vi "电信1801-2018012704-杜兴安-虚拟仪器作业3.vi"() -> ()   [LabVIEW 2020]
uses:
  <vilib>/Native 3D Graph/xcontrol/3DPC_SurfacePlot.xctl
  <vilib>/Waveform/DWDTOps.llb/DWDT Binary U32 to Digital.vi
  <vilib>/Analysis/NI_AALBase.lvlib
  <vilib>/Native 3D Graph/classes/Base Datatype.lvclass
panel:
  out "3D Graph 7":refnum<class "Base Datatype.lvclass">[](xcontrol) caption="三维图形"
  out "波形图表 2":dbl[][](graph)
  out "数字波形图 2":digitalwaveform(graph)
  out "3D Graph 4":refnum<class "Base Datatype.lvclass">[](xcontrol) caption="三维图形"
  out "强度图 2":dbl[][](graph)
  out "XY图 2":cluster{dbl[], dbl[]}(graph)
  in  "界限值":dbl
  out "报警tip":bool
  out "温度计1":dbl(slide) scale=0.0..100.0
  in  "停止 3":bool
  out "电压显示":dbl
  in  "电压表":dbl(knob) scale=0.0..10.0
  in  "停止 2":bool
  out "波形图表":dbl[][](graph)
  out "数字波形图":digitalwaveform(graph)
  out "3D Graph 3":refnum<class "Base Datatype.lvclass">[](xcontrol) caption="三维图形"
  out "3D Graph 2":refnum<class "Base Datatype.lvclass">[](xcontrol) caption="三维图形"
  out "3D Graph":refnum<class "Base Datatype.lvclass">[](xcontrol) caption="三维图形"
  out "强度图":dbl[][](graph)
  out "XY图":cluster{dbl[], dbl[]}(graph)
  in  "?":bool
  out "报警提示":bool
  out "温度计":dbl(slide) scale=0.0..100.0
  in  "温度报警限值":dbl
  in  "电压表(V)":dbl(knob) scale=0.0..10.0
  out "电压值(V)":dbl
  in  "停止":bool
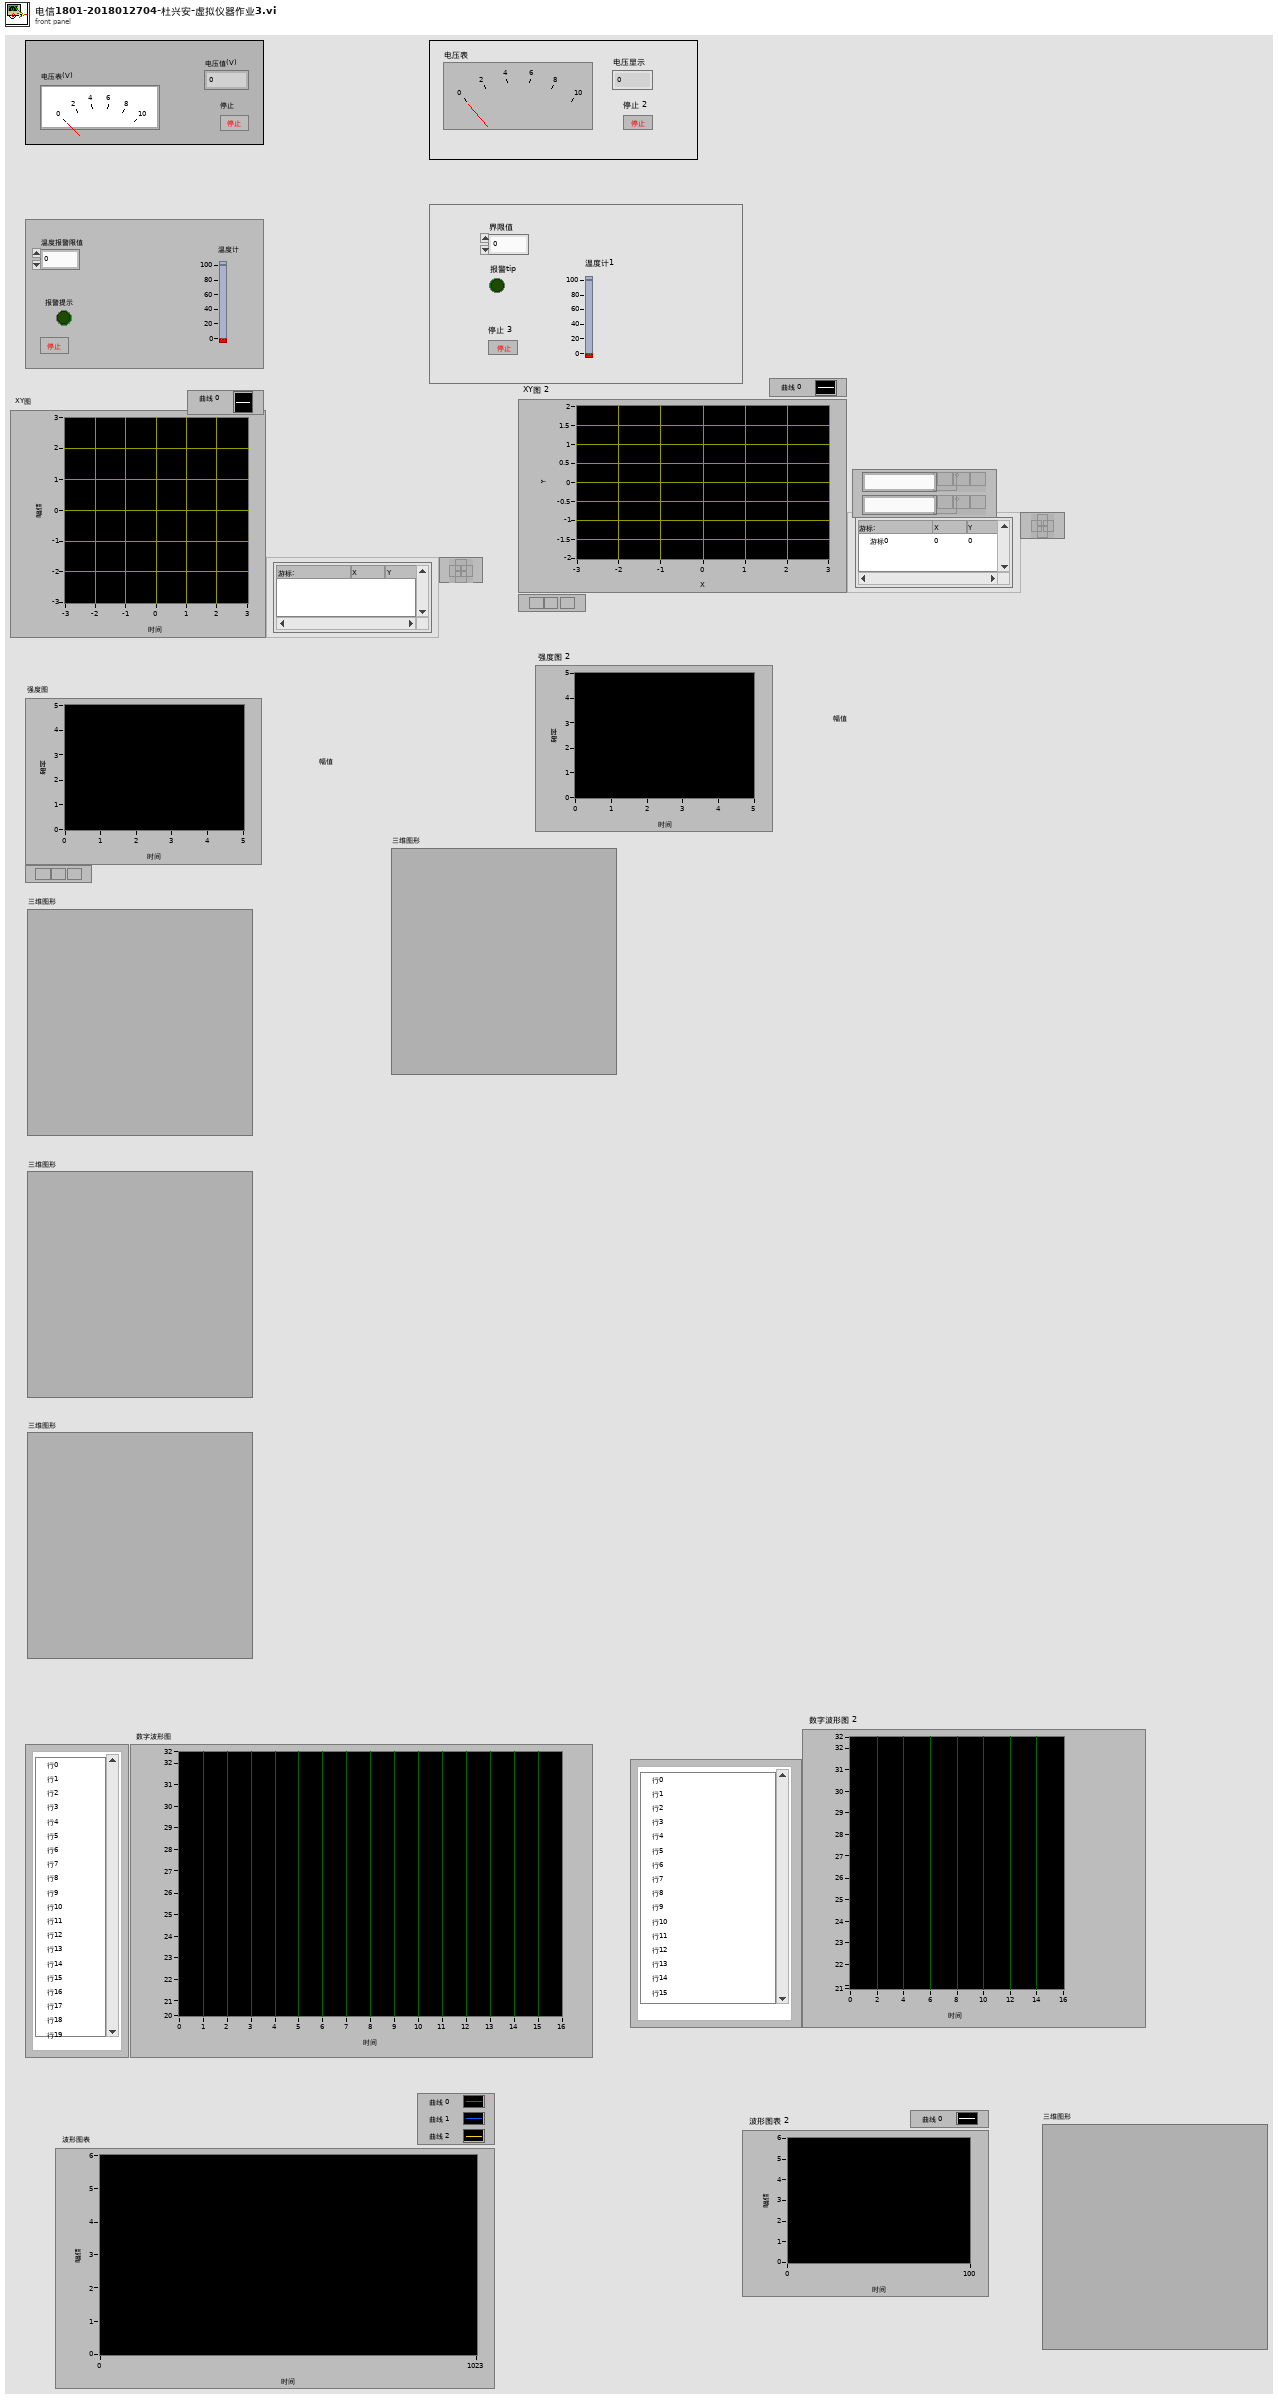
[diagram p1: front panel]
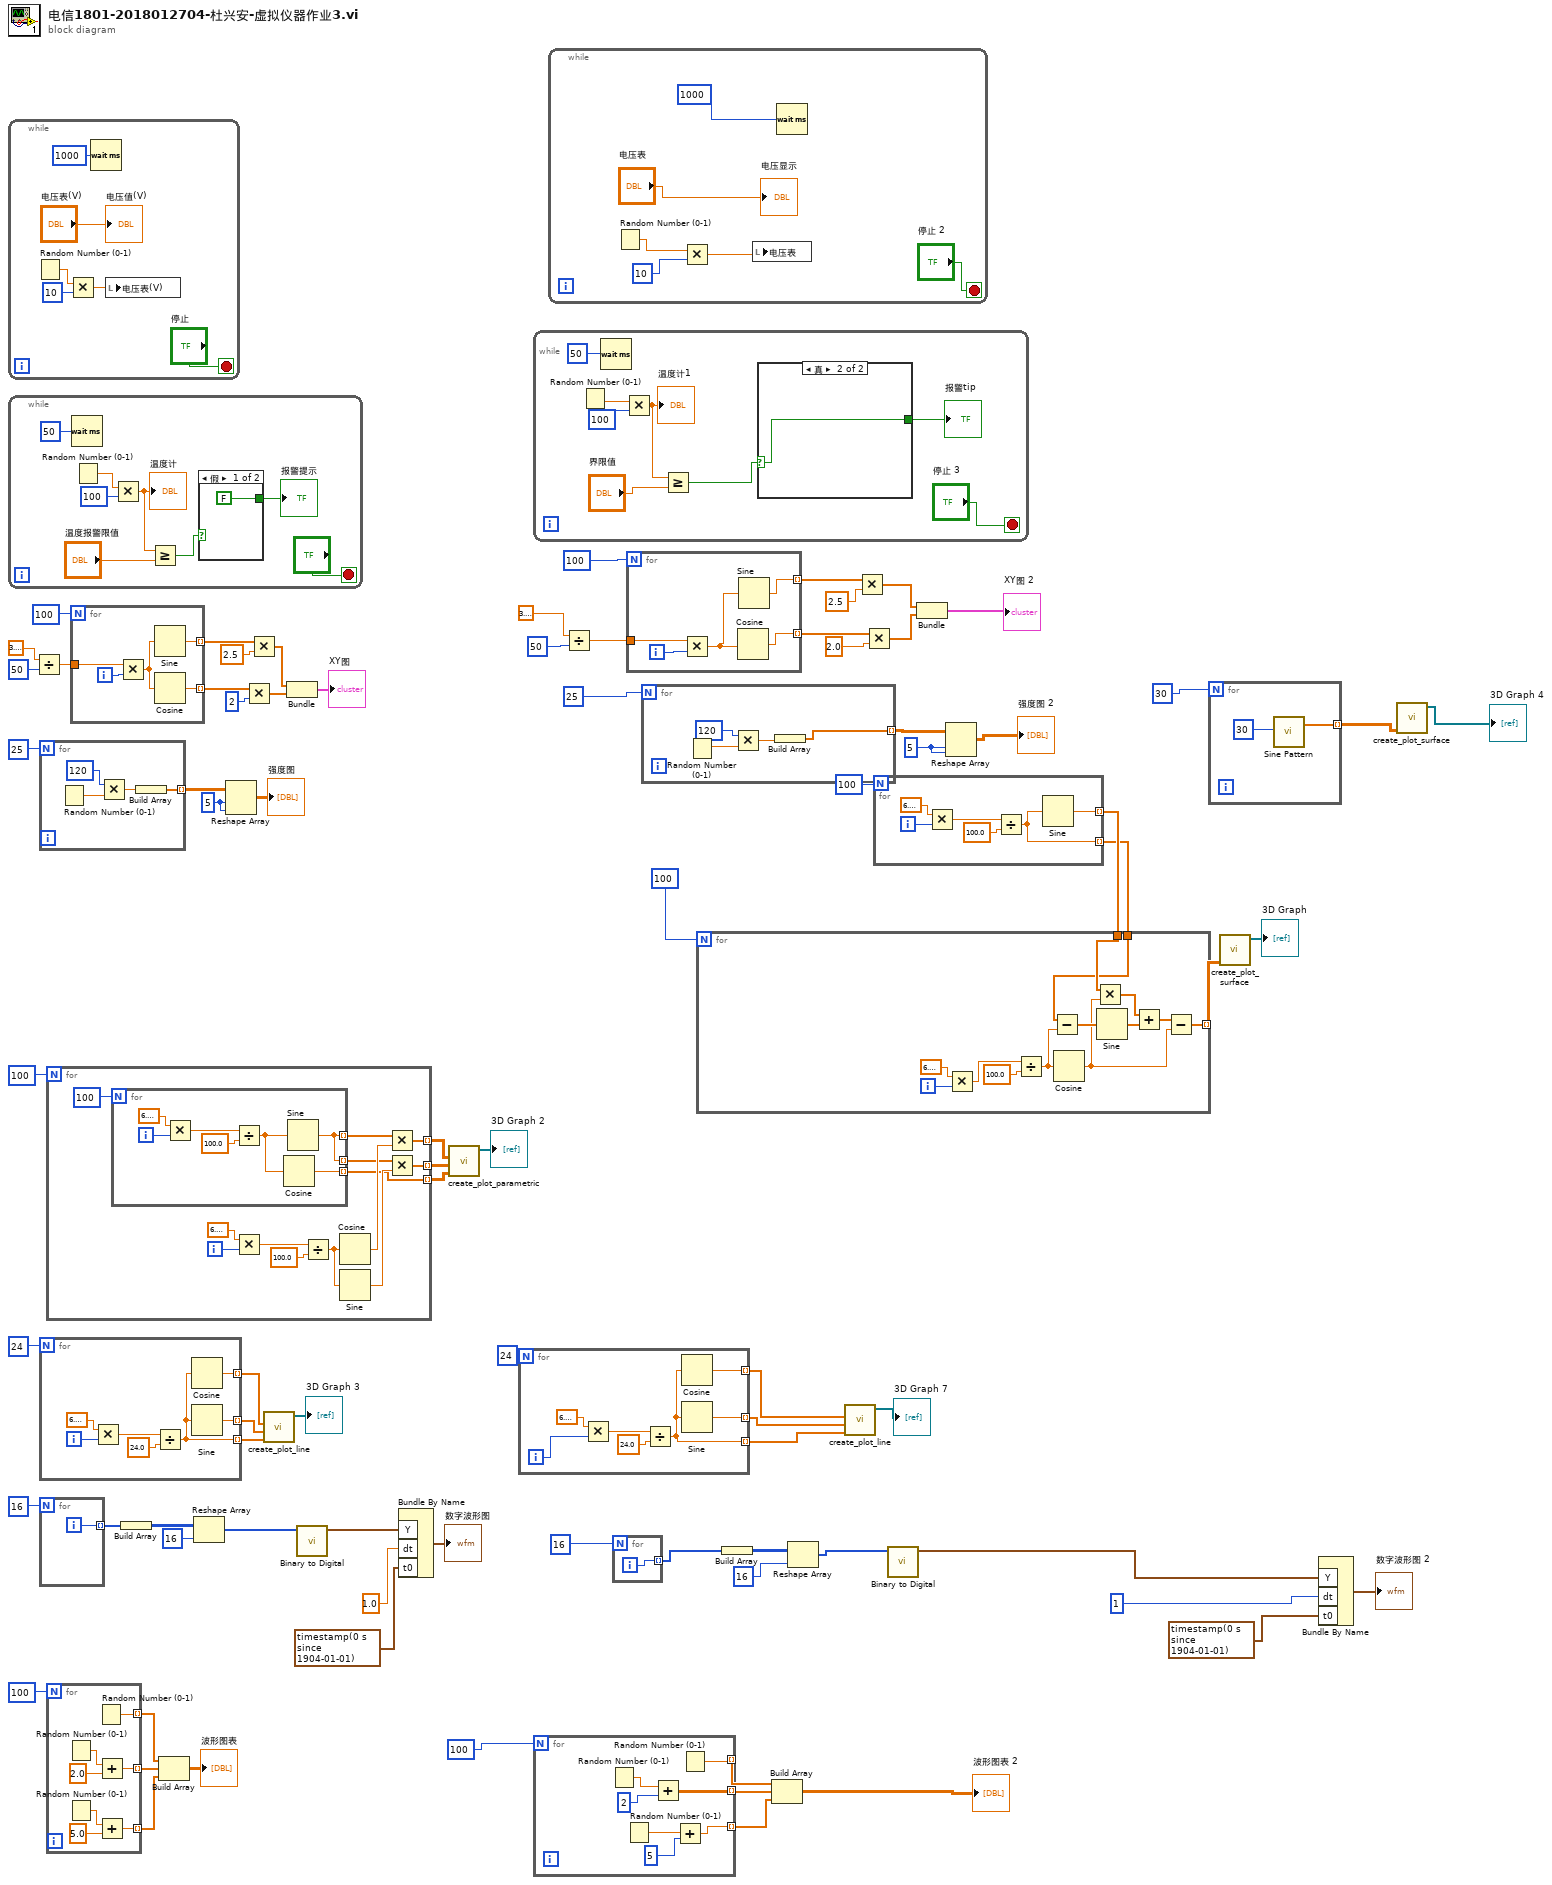
[diagram p0: block diagram]
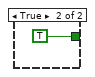
[diagram p3: hidden frame]
diagram:
  w27 = 5
  w68 = 5
  n1 = while {
    stop <- "停止" stop-if-true
    n2 = Random Number (0-1)() -> (number: 0 to 1=w87:dbl)
    n3 = Multiply(x=w87, y=10) -> (x*y=w85:dbl)
    n4 = Wait (ms)(milliseconds to wait=1000) -> ()  [unwired: 1 out]
    n5 = local write "电压表(V)"(w85) -> ()
    "电压值(V)" <- "电压表(V)"
  }
  n6 = while {
    stop <- "?" stop-if-true
    n7 = Wait (ms)(milliseconds to wait=50) -> ()  [unwired: 1 out]
    n8 = Random Number (0-1)() -> (number: 0 to 1=w94:dbl)
    n9 = Multiply(x=w94, y=100) -> (x*y=w92:dbl)
    "温度计" <- w92
    n10 = Greater Or Equal?(x=w92, y="温度报警限值") -> (x >= y?=w90:bool)
    n11 = case shown="假" w90 {
      tunnel: [FALSE TRUE] -> w91
      frame False {
      }
      frame True {
      }
    }
    "报警提示" <- w91
  }
  n12 = Divide(x=3.141592653589793, y=50) -> (x/y=w79:dbl)
  n13 = for {
    N: 25 -> [_]
    tunnel: [w102] -> w69 mode=indexing
    n14 = Random Number (0-1)() -> (number: 0 to 1=w99:dbl)
    n15 = Multiply(x=120, y=w99) -> (x*y=w100:dbl)
    n16 = Build Array(w100) -> (w102:dbl[])
  }
  n17 = for {
    N: 24 -> [_]
    tunnel: [w105] -> w57 mode=indexing
    tunnel: [w104] -> w56 mode=indexing
    tunnel: [w103] -> w55 mode=indexing
    i -> [w106]
    n18 = Multiply(x=6.283185307179586, y=w106) -> (x*y=w109:dbl)
    n19 = Divide(x=w109, y=24.0) -> (x/y=w103:dbl)
    n20 = Cosine(x=w103) -> (cos(x)=w105:dbl)
    n21 = Sine(x=w103) -> (sin(x)=w104:dbl)
  }
  n22 = for {
    N: 16 -> [_]
    tunnel: [w110] -> w53 mode=indexing
    i -> [w110]
  }
  n23 = for {
    N: 100 -> [_]
    tunnel: [w113] -> w62 mode=indexing
    tunnel: [w112] -> w61 mode=indexing
    tunnel: [w111] -> w60 mode=indexing
    i -> [w122]
    n24 = for {
      N: 100 -> [_]
      tunnel: [w125] -> w117 mode=indexing
      tunnel: [w125] -> w115 mode=indexing
      tunnel: [w124] -> w113 mode=indexing
      i -> [w127]
      n25 = Multiply(x=6.283185307179586, y=w127) -> (x*y=w130:dbl)
      n26 = Divide(x=w130, y=100.0) -> (x/y=w126:dbl)
      n27 = Cosine(x=w126) -> (cos(x)=w124:dbl)
      n28 = Sine(x=w126) -> (sin(x)=w125:dbl)
    }
    n29 = Multiply(x=6.283185307179586, y=w122) -> (x*y=w119:dbl)
    n30 = Divide(x=w119, y=100.0) -> (x/y=w118:dbl)
    n31 = Cosine(x=w118) -> (cos(x)=w116:dbl)
    n32 = Sine(x=w118) -> (sin(x)=w114:dbl)
    n33 = Multiply(x=w117, y=w116) -> (x*y=w112:dbl[])
    n34 = Multiply(x=w115, y=w114) -> (x*y=w111:dbl[])
  }
  n35 = for {
    N: 100 -> [_]
    tunnel: [w133] -> w44 mode=indexing
    tunnel: [w132] -> w43 mode=indexing
    tunnel: [w131] -> w42 mode=indexing
    n36 = Random Number (0-1)() -> (number: 0 to 1=w137:dbl)
    n37 = Random Number (0-1)() -> (number: 0 to 1=w135:dbl)
    n38 = Random Number (0-1)() -> (number: 0 to 1=w133:dbl)
    n39 = Add(x=w137, y=2.0) -> (x+y=w132:dbl)
    n40 = Add(x=w135, y=5.0) -> (x+y=w131:dbl)
  }
  n41 = for {
    N: 100 -> [_]
    tunnel: w79 -> [w141]
    tunnel: [w139] -> w74 mode=indexing
    tunnel: [w138] -> w75 mode=indexing
    i -> [w142]
    n42 = Multiply(x=w141, y=w142) -> (x*y=w140:dbl)
    n43 = Sine(x=w140) -> (sin(x)=w139:dbl)
    n44 = Cosine(x=w140) -> (cos(x)=w138:dbl)
  }
  n45 = Build Array(w53) -> (w51:i32[][])
  n46 = Build Array(w44, w43, w42) -> (→"波形图表":dbl[][])
  n47 = Reshape Array(w51, 16) -> (w46:i32[])
  n48 = Reshape Array(w69, w68, w68) -> (→"强度图":dbl[][])
  n49 = Multiply(x=w75, y=2) -> (x*y=w72:dbl[])
  n50 = Multiply(x=w74, y=2.5) -> (x*y=w73:dbl[])
  n51 = call <vilib>:"create_plot_line.vi"("z vector"=w55, "y vector"=w56, "x vector"=w57) -> ("plots out"=→"3D Graph 3":refnum<class "Base Datatype.lvclass">[])  [unwired: 2 in, 6 out]
  n52 = Bundle(w73, w72) -> (→"XY图":cluster{dbl[], dbl[]})  [unwired: 1 in]
  n53 = call-poly <vilib>:"Binary to Digital.vi"("binary array"=w46) -> ("digital waveform"=w50:digitalwaveform)  [unwired: 9 in, 1 out]
  n54 = Bundle By Name ("创建波形")("Y"=w50, "dt"=1.0, "t0"=timestamp(0 s since 1904-01-01)) -> (→"数字波形图":digitalwaveform)  [unwired: 1 in]
  n55 = call <vilib>:"create_plot_parametric.vi"("z matrix"=w62, "y matrix"=w60, "x matrix"=w61) -> ("plots out"=→"3D Graph 2":refnum<class "Base Datatype.lvclass">[])  [unwired: 2 in, 6 out]
  n56 = for {
    N: 24 -> [_]
    tunnel: [w146] -> w6 mode=indexing
    tunnel: [w145] -> w5 mode=indexing
    tunnel: [w144] -> w4 mode=indexing
    i -> [w143]
    n57 = Multiply(x=6.283185307179586, y=w143) -> (x*y=w149:dbl)
    n58 = Divide(x=w149, y=24.0) -> (x/y=w146:dbl)
    n59 = Cosine(x=w146) -> (cos(x)=w144:dbl)
    n60 = Sine(x=w146) -> (sin(x)=w145:dbl)
  }
  n61 = while {
    stop <- "停止 3" stop-if-true
    n62 = Random Number (0-1)() -> (number: 0 to 1=w155:dbl)
    n63 = Wait (ms)(milliseconds to wait=50) -> ()  [unwired: 1 out]
    n64 = Multiply(x=w155, y=100) -> (x*y=w153:dbl)
    "温度计1" <- w153
    n65 = Greater Or Equal?(x=w153, y="界限值") -> (x >= y?=w151:bool)
    n66 = case shown="真" w151 {
      selector: w151 -> [w158 w159]
      tunnel: [w158 w159] -> w150
      frame False {
      }
      frame True {
      }
    }
    "报警tip" <- w150
  }
  n67 = for {
    N: 100 -> [_]
    tunnel: [w166] -> w9 mode=indexing
    tunnel: [w161] -> w10 mode=indexing
    tunnel: [w160] -> w11 mode=indexing
    n68 = Random Number (0-1)() -> (number: 0 to 1=w162:dbl)
    n69 = Random Number (0-1)() -> (number: 0 to 1=w165:dbl)
    n70 = Add(x=w162, y=2) -> (x+y=w161:dbl)
    n71 = Add(x=w165, y=5) -> (x+y=w160:dbl)
    n72 = Random Number (0-1)() -> (number: 0 to 1=w166:dbl)
  }
  n73 = while {
    stop <- "停止 2" stop-if-true
    n74 = Random Number (0-1)() -> (number: 0 to 1=w170:dbl)
    n75 = Multiply(x=w170, y=10) -> (x*y=w168:dbl)
    n76 = local write "电压表"(w168) -> ()
    n77 = Wait (ms)(milliseconds to wait=1000) -> ()  [unwired: 1 out]
    "电压显示" <- "电压表"
  }
  n78 = Divide(x=3.141592653589793, y=50) -> (x/y=w38:dbl)
  n79 = for {
    N: 16 -> [_]
    tunnel: [w173] -> w20 mode=indexing
    i -> [w173]
  }
  n80 = for {
    N: 100 -> [_]
    tunnel: w38 -> [w177]
    tunnel: [w175] -> w37 mode=indexing
    tunnel: [w174] -> w36 mode=indexing
    i -> [w178]
    n81 = Multiply(x=w177, y=w178) -> (x*y=w176:dbl)
    n82 = Cosine(x=w176) -> (cos(x)=w174:dbl)
    n83 = Sine(x=w176) -> (sin(x)=w175:dbl)
  }
  n84 = for {
    N: 25 -> [_]
    tunnel: [w179] -> w28 mode=indexing
    n85 = Random Number (0-1)() -> (number: 0 to 1=w181:dbl)
    n86 = Multiply(x=120, y=w181) -> (x*y=w180:dbl)
    n87 = Build Array(w180) -> (w179:dbl[])
  }
  n88 = Build Array(w20) -> (w19:i32[][])
  n89 = Build Array(w9, w10, w11) -> (→"波形图表 2":dbl[][])
  n90 = Reshape Array(w19, 16) -> (w17:i32[])
  n91 = call <vilib>:"create_plot_line.vi"("z vector"=w6, "y vector"=w5, "x vector"=w4) -> ("plots out"=→"3D Graph 7":refnum<class "Base Datatype.lvclass">[])  [unwired: 2 in, 6 out]
  n92 = Multiply(x=w37, y=2.5) -> (x*y=w33:dbl[])
  n93 = Multiply(x=w36, y=2.0) -> (x*y=w32:dbl[])
  n94 = for {
    N: 100 -> [_]
    tunnel: [w184] -> w2 mode=indexing
    tunnel: [w183] -> w1 mode=indexing
    i -> [w187]
    n95 = Multiply(x=6.283185307179586, y=w187) -> (x*y=w186:dbl)
    n96 = Divide(x=w186, y=100.0) -> (x/y=w183:dbl)
    n97 = Sine(x=w183) -> (sin(x)=w184:dbl)
  }
  n98 = for {
    N: 100 -> [_]
    tunnel: [w191] -> w65 mode=indexing
    tunnel: w2 -> [w190]
    tunnel: w1 -> [w189]
    i -> [w198]
    n99 = Multiply(x=6.283185307179586, y=w198) -> (x*y=w200:dbl)
    n100 = Divide(x=w200, y=100.0) -> (x/y=w196:dbl)
    n101 = Subtract(x=w189, y=w196) -> (x-y=w197:dbl[])
    n102 = Cosine(x=w196) -> (cos(x)=w192:dbl)
    n103 = Multiply(x=w190, y=w192) -> (x*y=w195:dbl[])
    n104 = Sine(x=w197) -> (sin(x)=w194:dbl[])
    n105 = Add(x=w195, y=w194) -> (x+y=w193:dbl[])
    n106 = Subtract(x=w193, y=w192) -> (x-y=w191:dbl[])
  }
  n107 = call-poly <vilib>:"Binary to Digital.vi"("binary array"=w17) -> ("digital waveform"=w16:digitalwaveform)  [unwired: 9 in, 1 out]
  n108 = Bundle(w33, w32) -> (→"XY图 2":cluster{dbl[], dbl[]})  [unwired: 1 in]
  n109 = Reshape Array(w28, w27, w27) -> (→"强度图 2":dbl[][])
  n110 = for {
    N: 30 -> [_]
    tunnel: [w202] -> w24 mode=indexing
    n111 = call <vilib>:"Sine Pattern.vi"("amplitude"=30) -> ("Sinusoidal Pattern"=w202:dbl[])  [unwired: 3 in, 1 out]
  }
  n112 = call <vilib>:"create_plot_surface.vi"("z matrix"=w65) -> ("plots out"=→"3D Graph":refnum<class "Base Datatype.lvclass">[])  [unwired: 4 in, 6 out]
  n113 = Bundle By Name ("创建波形")("Y"=w16, "dt"=1, "t0"=timestamp(0 s since 1904-01-01)) -> (→"数字波形图 2":digitalwaveform)  [unwired: 1 in]
  n114 = call <vilib>:"create_plot_surface.vi"("z matrix"=w24) -> ("plots out"=→"3D Graph 4":refnum<class "Base Datatype.lvclass">[])  [unwired: 4 in, 6 out]
